vi "Initialize.vi"(8 "error in (no error)":errorcluster, 11 "InferenceTCP in":refnum<class "InferenceTCP.lvclass">) -> (0 "error out":errorcluster, 3 "InferenceTCP out":refnum<class "InferenceTCP.lvclass">)   [LabVIEW 2019, in "InferenceTCP.lvlib" / "InferenceTCP.lvclass"]
uses:
  InferenceTCP.lvclass
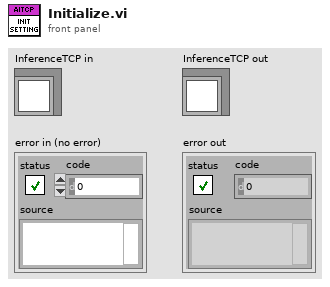
[diagram p1: front panel]
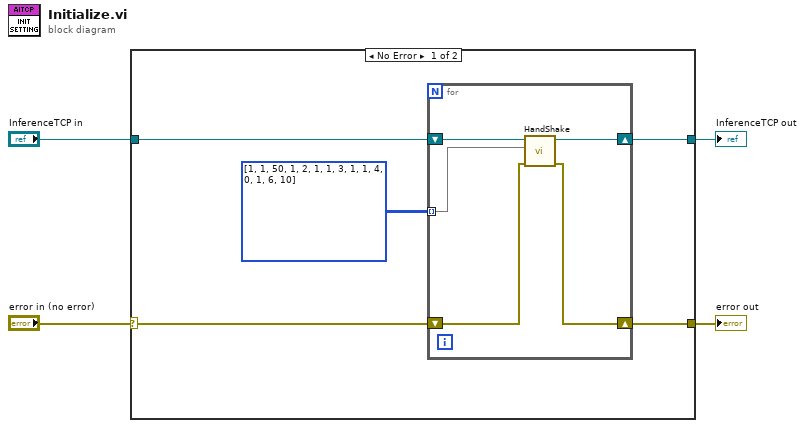
[diagram p0: block diagram]
diagram:
  n1 = case shown="No Error" "error in (no error)" {
    selector: "error in (no error)" -> [w6 w16]
    tunnel: [w8 w16] -> w3
    tunnel: [w7 w15] -> w1
    tunnel: "InferenceTCP in" -> [w5 w15]
    frame No Error {
      n2 = for {
        shift-right: [w12] -> w7
        shift-left: w5 -> [w14]
        tunnel: u8[][] [[1, 1, 50], [1, 2, 1], [1, 3, 1], [1, 4, 0], [1, 6, 10]] -> [w13] mode=indexing
        shift-right: [w10] -> w8
        shift-left: w6 -> [w11]
        n3 = call "HandShake.vi"("error in (no error)"=w11, "Data In"=w13, "InferenceTCP in"=w14) -> ("error out"=w10:errorcluster, "InferenceTCP out"=w12:refnum<class "InferenceTCP.lvclass">)  [unwired: 6 in, 1 out]
      }
    }
    frame Error {
    }
  }
  "error out" <- w3
  "InferenceTCP out" <- w1
